vi "Disconnect.vi"(8 "error in (no error)":errorcluster, 11 "AF Queue Stream in":refnum<class "AF Queue Stream.lvclass">) -> (0 "error out":errorcluster, 3 "AF Queue Stream out":refnum<class "AF Queue Stream.lvclass">)   [LabVIEW 2020, in "AF Queue Stream.lvclass"]
doc: "Override this method to specify the action the local copy of this object will perform to disconnect from its remote counterpart."
uses:
  AF Queue Stream.lvclass
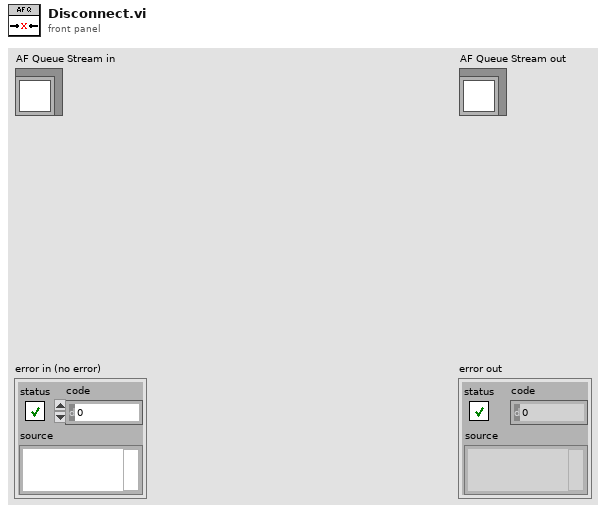
[diagram p1: front panel]
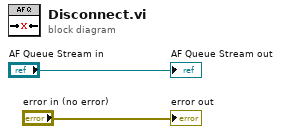
[diagram p0: block diagram]
diagram:
  "error out" <- "error in (no error)"
  "AF Queue Stream out" <- "AF Queue Stream in"
